vi "Get Downloads.vi"(8 "error in (no error)":errorcluster, 11 "Package in":refnum<class "Package.lvclass">) -> (0 "error out":errorcluster, 2 "Downloads":i32, 3 "Package out":refnum<class "Package.lvclass">)   [LabVIEW 2020, in "GCentral-API.lvlib" / "Package.lvclass"]
uses:
  Package.lvclass
  Package.lvclass/Package.ctl
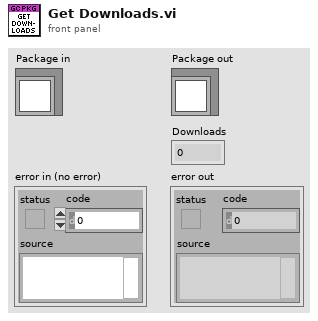
[diagram p1: front panel]
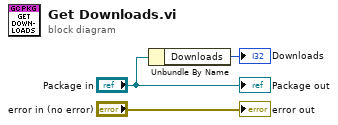
[diagram p0: block diagram]
diagram:
  n1 = Unbundle By Name("Package in") -> ("Downloads"=→"Downloads":i32)
  "error out" <- "error in (no error)"
  "Package out" <- "Package in"
